vi "Built In Homing Function - All Axis.vi"(2 "Error In":errorcluster, 3 "Home":bool, 4 "Reference In":refnum<class "_Controller.lvclass">) -> (0 "Error Out":errorcluster, 1 "Reference Out":refnum<class "_Controller.lvclass">)   [LabVIEW 2020]
doc: "Moves the machine to its home position which is defined by the physical triggers on the machines. Need to indicate the direction as there are triggers on each corner of the machine.\n\nArgs:\n\nReference In: Incoming communication (reference) between LabView and the scanning rig controller\nError In: Checks for any errors with the incoming communication (reference)\n\nReturns:\n\nReference Out: Output communnication (reference) between LabView and controller\nError Out: Checks for any error with output communication (reference)"
uses:
  <instrlib>/Arcus Ethernet Driver 1.0.0/ArcusEthernetComm/classes/Controller/_Controller.lvclass
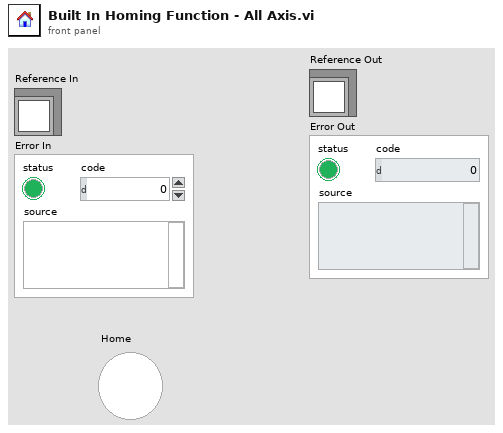
[diagram p1: front panel]
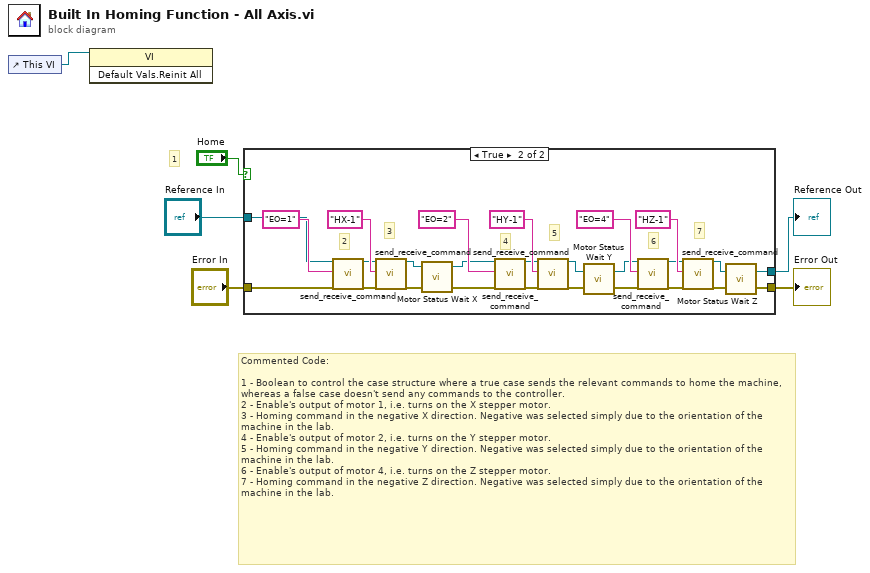
[diagram p0: block diagram]
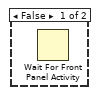
[diagram p2: hidden frame]
diagram:
  # "Commented Code:\n\n1 - Boolean to control the case structure where a true case sends the relevant commands to home the machine, whereas a false case doesn't send any commands to the controller.\n2 - Enable's output of motor 1, i.e. turns on the X stepper motor.\n3 - Homing command in the negative X direction. Negative was selected simply due to the orientation of the machine in the lab.\n4 - Enable's output of motor 2, i.e. turns on the Y stepper motor.\n5 - Homing command in the negative Y direction. Negative was selected simply due to the orientation of the machine in the lab.\n6 - Enable's output of motor 4, i.e. turns on the Z stepper motor.\n7 - Homing command in the negative Z direction. Negative was selected simply due to the orientation of the machine in the lab."
  # "1"
  n1 = control-ref of="This VI"() -> (w1:refnum<vi>)
  n2 = invoke class="VI" method="Default Vals.Reinit All"(reference=w1) -> ()  [unwired: 2 in, 3 out]
  n3 = case shown="True" "Home" {
    tunnel: "Reference In" -> [_ w12]
    tunnel: "Error In" -> [_ w11]
    tunnel: [_ w7] -> w2
    tunnel: [_ w8] -> w5
    frame False {
      n4 = Wait For Front Panel Activity() -> ()  [unwired: 3 in, 1 out]
    }
    frame True {
      # "7"
      # "6"
      # "5"
      # "4"
      # "3"
      # "2"
      n5 = call <instrlib>:"send_receive_command.vi"("reference (in)"=w12, "ASCII Command (in)"="EO=1", "error in (no error)"=w11) -> ("reference (out)"=w20:refnum<class "_Controller.lvclass">, "error out"=w19:errorcluster)  [unwired: 12 in, 3 out]
      n6 = call <instrlib>:"send_receive_command.vi"("reference (in)"=w20, "ASCII Command (in)"="HX-1", "error in (no error)"=w19) -> ("reference (out)"=w29:refnum<class "_Controller.lvclass">, "error out"=w28:errorcluster)  [unwired: 12 in, 3 out]
      n7 = call "Motor Status Wait X.vi"("Error In"=w28, "Reference In"=w29) -> ("Error Out"=w18:errorcluster, "Reference Out"=w17:refnum<class "_Controller.lvclass">)  [unwired: 2 in]
      n8 = call <instrlib>:"send_receive_command.vi"("reference (in)"=w17, "ASCII Command (in)"="EO=2", "error in (no error)"=w18) -> ("reference (out)"=w25:refnum<class "_Controller.lvclass">, "error out"=w24:errorcluster)  [unwired: 12 in, 3 out]
      n9 = call <instrlib>:"send_receive_command.vi"("reference (in)"=w25, "ASCII Command (in)"="HY-1", "error in (no error)"=w24) -> ("reference (out)"=w16:refnum<class "_Controller.lvclass">, "error out"=w15:errorcluster)  [unwired: 12 in, 3 out]
      n10 = call "Motor Status Wait Y.vi"("Error In"=w15, "Reference In"=w16) -> ("Error Out"=w14:errorcluster, "Reference Out"=w13:refnum<class "_Controller.lvclass">)
      n11 = call <instrlib>:"send_receive_command.vi"("reference (in)"=w13, "ASCII Command (in)"="EO=4", "error in (no error)"=w14) -> ("reference (out)"=w22:refnum<class "_Controller.lvclass">, "error out"=w21:errorcluster)  [unwired: 12 in, 3 out]
      n12 = call <instrlib>:"send_receive_command.vi"("reference (in)"=w22, "ASCII Command (in)"="HZ-1", "error in (no error)"=w21) -> ("reference (out)"=w10:refnum<class "_Controller.lvclass">, "error out"=w9:errorcluster)  [unwired: 12 in, 3 out]
      n13 = call "Motor Status Wait Z.vi"("Error In"=w9, "Reference In"=w10) -> ("Error Out"=w7:errorcluster, "Reference Out"=w8:refnum<class "_Controller.lvclass">)
    }
  }
  "Reference Out" <- w5
  "Error Out" <- w2
